vi "GetXbox.vi"() -> (1 "Data Out":T1)   [LabVIEW 2017]
uses:
  C:/Windows/System32/XInput9_1_0.dll
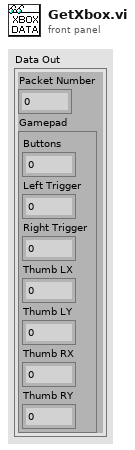
[diagram p1: front panel]
types:
  T1 = cluster{"Packet Number":u32, "Gamepad":cluster{"Buttons":u16, "Left Trigger":u8, "Right Trigger":u8, "Thumb LX":i16, "Thumb LY":i16, "Thumb RX":i16, "Thumb RY":i16}}
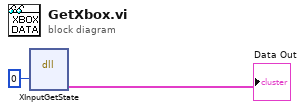
[diagram p0: block diagram]
diagram:
  n1 = dll-call lib="C:/Windows/System32/XInput9_1_0.dll" fn="XInputGetState"("dwUserIndex"=u32 0) -> ("Data Out"=→"Data Out":T1)  [unwired: 6 in, 2 out]
